vi "GEA2 to LEUI.vi"(0 "LEUI_LEDs_In":T1, 7 "Raw Data In":string) -> (8 "LEUI_LEDs_Out":T1)   [LabVIEW 2014]
uses:
  type defs/LEUI_LEDs_SLB.ctl
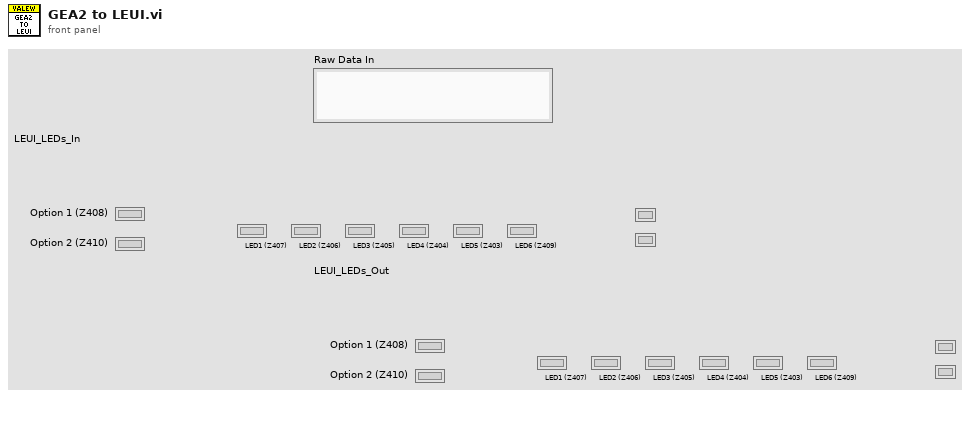
[diagram p1: front panel]
types:
  T1 = typedef "LEUI_LEDs_SLB.ctl" = cluster{"Pause (Z401)":bool, "Lid Locked (Z402)":bool, "LED1 (Z407)":bool, "LED2 (Z406)":bool, "LED3 (Z405)":bool, "LED4 (Z404)":bool, "LED5 (Z403)":bool, "LED6 (Z409)":bool, "Option 1 (Z408)":bool, "Option 2 (Z410)":bool}
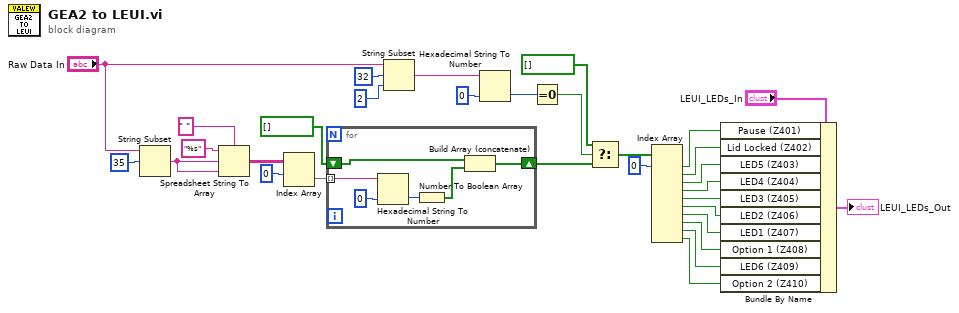
[diagram p0: block diagram]
diagram:
  n1 = String Subset(string="Raw Data In", offset (0)=35) -> (substring=w24:string)  [unwired: 1 in]
  n2 = Spreadsheet String To Array(delimiter (Tab)=" ", format string="%s", spreadsheet string=w24, array type (2D Dbl)=w24) -> (array=w28:string[][])
  n3 = Index Array(array=w28, index (row)=0) -> (element=w25:string[])  [unwired: 1 in]
  n4 = for {
    tunnel: w25 -> [w37] mode=indexing
    shift-right: [w33] -> w17
    shift-left: bool[] [] -> [w35]
    n5 = Hexadecimal String To Number(string=w37, default (0uL)=u8 0) -> (number=w36:u8)  [unwired: 1 in, 1 out]
    n6 = Number To Boolean Array(number=w36) -> (Boolean array=w34:bool[])
    n7 = Build Array (concatenate)(w35, w34) -> (w33:bool[])
  }
  n8 = String Subset(string="Raw Data In", offset (0)=32, length (rest)=2 ("length (rest)")) -> (substring=w21:string)
  n9 = Hexadecimal String To Number(string=w21, default (0uL)=u32 0 ("default (0 U32)")) -> (number=w19:u32)  [unwired: 1 in, 1 out]
  n10 = Equal To 0?(x=w19) -> (x = 0?=w18:bool)
  n11 = Select(t=bool[] [], s=w18, f=w17) -> (s? t:f=w15:bool[])
  n12 = Index Array(array=w15, index #1=0 ("index")) -> (element #1=w14:bool, element #2=w6:bool, element #3=w11:bool, element #4=w10:bool, element #5=w9:bool, element #6=w8:bool, element #7=w7:bool, element #8=w5:bool, element #9=w4:bool, element #10=w3:bool)  [unwired: 9 in]
  n13 = Bundle By Name(cluster="LEUI_LEDs_In", "Pause (Z401)"=w14, "Lid Locked (Z402)"=w6, "LED5 (Z403)"=w11, "LED4 (Z404)"=w10, "LED3 (Z405)"=w9, "LED2 (Z406)"=w8, "LED1 (Z407)"=w7, "Option 1 (Z408)"=w5, "LED6 (Z409)"=w4, "Option 2 (Z410)"=w3) -> (→"LEUI_LEDs_Out":T1)
